vi "MoveStage.vi"(5 "calbration (um/step)":dbl, 6 "stepPolarity":dbl, 7 "stepSize (mm)":dbl, 8 "error in (no error)":errorcluster, 9 "controllerAddress":i32=1, 10 "ChannelNumber":i32=1, 11 "reference":refnum<k24>) -> (0 "error out":errorcluster, 3 "reference out":refnum<k24>)   [LabVIEW 2013]
uses:
  C:/GEECS/Developers Version/builds/Device builds/AgilisPiezoStage/AgilisCmdLib.dll
  AgilisCmdLib.dll
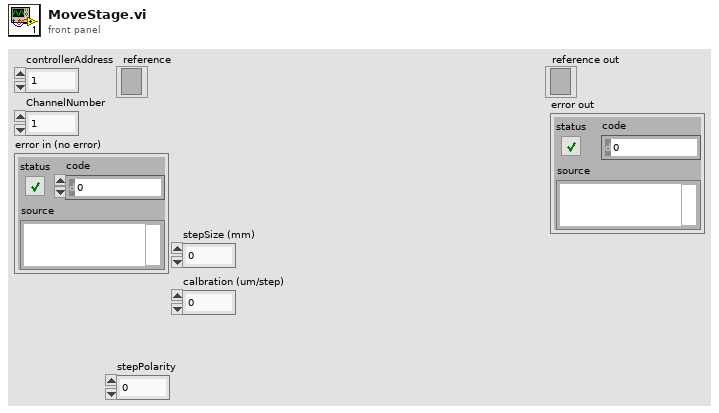
[diagram p1: front panel]
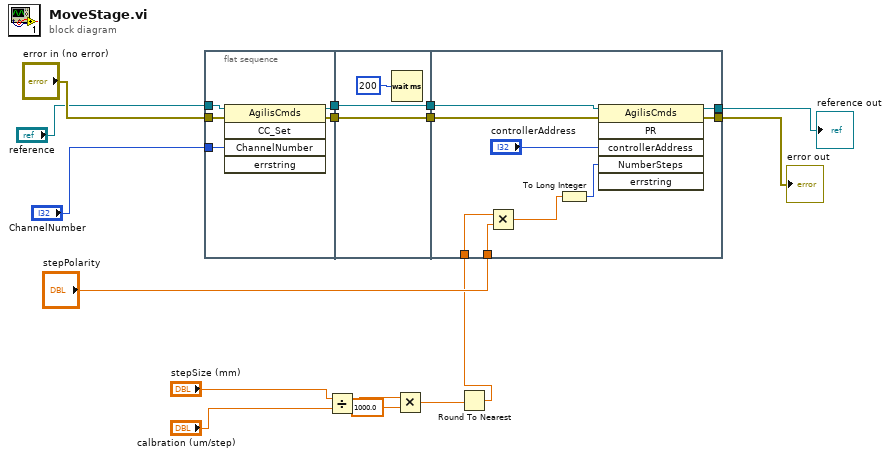
[diagram p0: block diagram]
diagram:
  n1 = flat-sequence {
    tunnel: [w21] -> w16
    tunnel: [w20] -> w15
    tunnel: "error in (no error)" -> [w19]
    tunnel: "reference" -> [w18]
    tunnel: "ChannelNumber" -> [w17]
    tunnel: w16 -> [w23]
    tunnel: w15 -> [w22]
    tunnel: [w23] -> w14
    tunnel: [w22] -> w13
    tunnel: w14 -> [w31]
    tunnel: w13 -> [w30]
    tunnel: [w29] -> w9
    tunnel: [w28] -> w8
    tunnel: "stepPolarity" -> [w27]
    tunnel: w1 -> [w25]
    frame #0 {
      n2 = invoke class="AgilisCmds" method="CC_Set"(reference=w18, error in=w19, "ChannelNumber"=w17) -> (reference out=w21:refnum<k24>, error out=w20:errorcluster)  [unwired: 2 in, 3 out]
    }
    frame #1 {
      n3 = Wait (ms)(milliseconds to wait=u32 200) -> ()  [unwired: 1 out]
    }
    frame #2 {
      n4 = Multiply(x=w25, y=w27) -> (x*y=w26:dbl)
      n5 = To Long Integer(number=w26) -> (32bit integer=w32:i32)
      n6 = invoke class="AgilisCmds" method="PR"(reference=w31, error in=w30, "controllerAddress"="controllerAddress", "NumberSteps"=w32) -> (reference out=w29:refnum<k24>, error out=w28:errorcluster)  [unwired: 2 in, 4 out]
    }
  }
  n7 = Divide(x="stepSize (mm)", y="calbration (um/step)") -> (x/y=w4:dbl)
  n8 = Multiply(x=w4, y=1000.0) -> (x*y=w2:dbl)
  n9 = Round To Nearest(number=w2) -> (nearest integer value=w1:dbl)
  "reference out" <- w9
  "error out" <- w8
